vi "JoysticksGlobal.vi"() -> ()   [LabVIEW 2014]
panel:
  out "Joysticks":T1
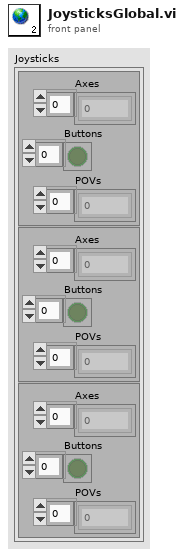
[diagram p1: front panel]
types:
  T1 = cluster{cluster{"Axes":dbl[], "Buttons":bool[], "POVs":i16[]}, cluster{"Axes":dbl[], "Buttons":bool[], "POVs":i16[]}, cluster{"Axes":dbl[], "Buttons":bool[], "POVs":i16[]}}
diagram:
